vi "Cryostation.Command Enum to String.vi"(8 "error in (no error)":errorcluster, 10 "Commands":T1, 11 "instrument.Cryostation in":refnum<class "instrument.Cryostation.lvclass">) -> (0 "error out":errorcluster, 1 "Commands []":string[](array[string]), 2 "Command":string, 3 "instrument.Cryostation out":refnum<class "instrument.Cryostation.lvclass">)   [LabVIEW 2016, in "instrument.Cryostation.lvclass"]
uses:
  instrument.Cryostation.lvclass
  Typedefs/Cryostation.Commands--enum.ctl
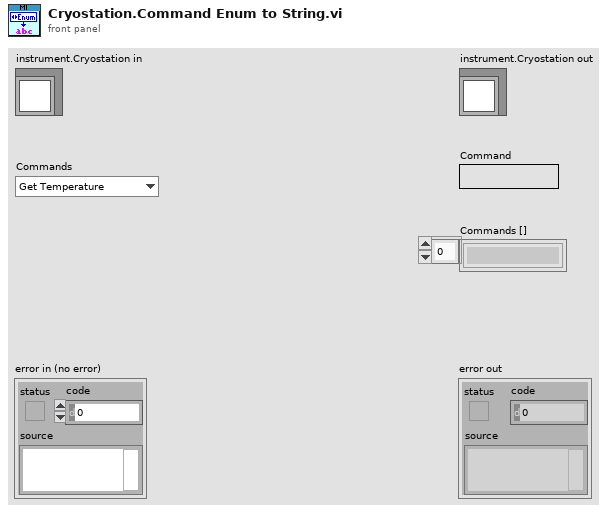
[diagram p1: front panel]
types:
  T1 = typedef "instrument.Cryostation.lvclass/Cryostation.Commands--enum.ctl" = enum16{"Get Temperature"}
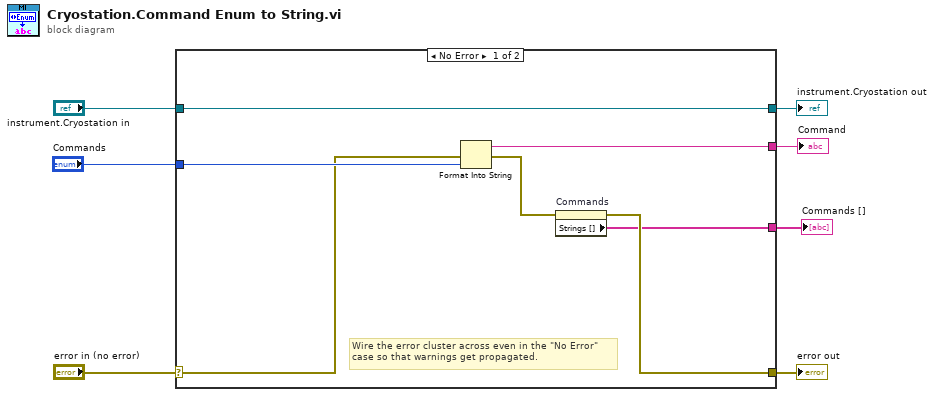
[diagram p0: block diagram]
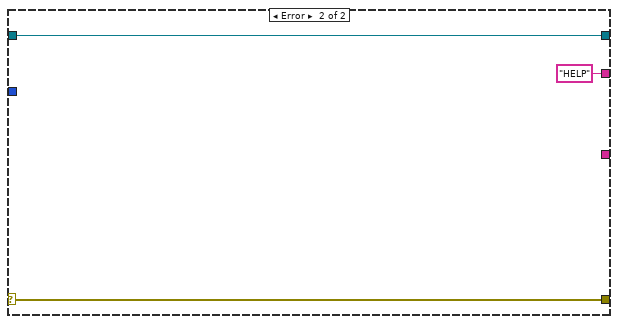
[diagram p2: hidden frame]
diagram:
  n1 = case shown="No Error" "error in (no error)" {
    selector: "error in (no error)" -> [w11 w17]
    tunnel: [w9 w17] -> w6
    tunnel: [w14 w16] -> w4
    tunnel: "instrument.Cryostation in" -> [w14 w16]
    tunnel: "Commands" -> [w13 _]
    tunnel: [w12 "HELP"] -> w2
    tunnel: [w8 _] -> w1
    frame No Error {
      # "Wire the error cluster across even in the \"No Error\"\ncase so that warnings get propagated."
      n2 = Format Into String(error in=w11, w13) -> (resulting string=w12:string, error out=w10:errorcluster)  [unwired: 2 in]
      n3 = property on="Commands" class="Enum (strict)"(error in=w10) -> (error out=w9:errorcluster, "Strings []"=w8:string[])  [unwired: 1 in, 1 out]
    }
    frame Error {
    }
  }
  "error out" <- w6
  "instrument.Cryostation out" <- w4
  "Command" <- w2
  "Commands []" <- w1
